vi "Log.vi"(8 "error in (no error)":errorcluster, 10 "Log Text":string, 11 "File Sink in":refnum<class "File Sink.lvclass">) -> (0 "error out":errorcluster, 3 "File Sink out":refnum<class "File Sink.lvclass">)   [LabVIEW 2025, in "LV Logging.lvlib" / "File Sink.lvclass"]
uses:
  File Sink.lvclass
  File Sink.lvclass/File Sink.ctl
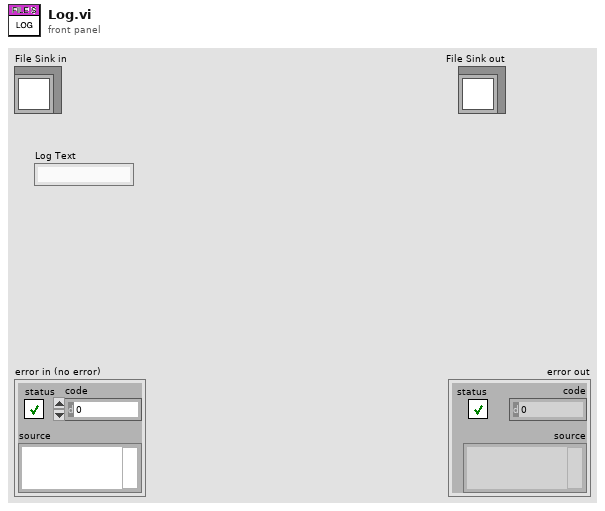
[diagram p1: front panel]
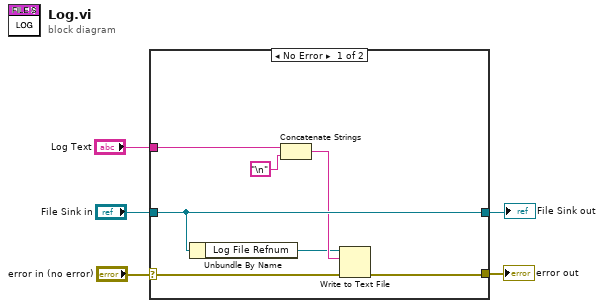
[diagram p0: block diagram]
diagram:
  n1 = case shown="No Error" "error in (no error)" {
    selector: "error in (no error)" -> [w11 w13]
    tunnel: [w10 w13] -> w4
    tunnel: [w12 w14] -> w3
    tunnel: "File Sink in" -> [w12 w14]
    tunnel: "Log Text" -> [w9 _]
    frame No Error {
      n2 = Unbundle By Name(w12) -> ("Log File Refnum"=w6:refnum<file>)
      n3 = Concatenate Strings(w9, "\n") -> (w8:string)
      n4 = Write to Text File(file (use dialog)=w6, text=w8, error in=w11) -> (error out=w10:errorcluster)  [unwired: 1 in, 2 out]
    }
    frame Error {
    }
  }
  "error out" <- w4
  "File Sink out" <- w3
